vi "Test Process Helper Loop Stopped when Process Stopped.vi"(8 "error in (no error)":errorcluster, 11 "Helper Loop Test In":refnum<class "Process Test.lvclass">) -> (0 "error out":errorcluster, 3 "Helper Loop Test Out":refnum<class "Process Test.lvclass">)   [LabVIEW 2020, in "Process Test.lvclass"]
uses:
  Process Test/Process Test.lvclass
  C:/Program Files (x86)/National Instruments/LabVIEW 2020/vi.lib/Asteme/LUnit/Test Case.lvclass
  Framework/Helper Loop/Helper Loop.lvclass
  <vilib>/Asteme/LUnit/Test Case.lvclass/Test Case.ctl
  <vilib>/Asteme/LUnit/LUnit Assertion Result.lvclass/LUnit Assertion Result.ctl
  Framework/Process/Process.lvclass/Process.ctl
  Support/Event Helpers/Dequeue Event Message by Message.vi
  <vilib>/Asteme/LUnit/Palette/Pass.vi
  <vilib>/Asteme/LUnit/Palette/Fail.vi
  <vilib>/Asteme/LUnit/Variant to string.vi
  <vilib>/Asteme/LUnit/Set Assertion Type.vi
  Framework/Process/Public/Get Lifecycle State.vi
  Framework/Process/Private/SubVIs/Wait for finish.vi
  Framework/Process/Protected/Messaging/Enqueue Message.vi
  Framework/Process/Private/SubVIs/Set Lifecycle State.vi
  <vilib>/Asteme/LUnit/Add test result.vi
  <vilib>/Asteme/LUnit/LUnit Get Test Case.vi
  <vilib>/Asteme/LUnit/LUnit Write Message.vi
  <vilib>/Asteme/LUnit/LUnit Write Description.vi
  <vilib>/Asteme/LUnit/LUnit Write Skipped.vi
  Support/Execution timer.vi
  <vilib>/Asteme/LUnit/LUnit Write Passed.vi
  <vilib>/Asteme/LUnit/LUnit Write Assertion Type.vi
  <vilib>/Utility/error.llb/Clear Errors.vi
  <vilib>/AdvancedString/1D String Array to Delimited String.vi
  <vilib>/Asteme/LUnit/Read Test Case Name.vi
  Support/Event Helpers/Dequeue Event Message.vi
  <vilib>/Asteme/LUnit/Assertion Result/LUnit Get Test Name.vi
  <vilib>/Utility/Data Type/Get Type Information.vi
  <vilib>/Utility/LVClass/Get LV Class Name.vi
  <vilib>/Utility/error.llb/Error Cluster From Error Code.vi
  <vilib>/Asteme/LUnit/LUnit Assertion Result.lvclass
  Framework/Process/Process.lvclass
  <vilib>/Asteme/LUnit/Test Case.lvclass
  Support/Event Helpers/Event Helpers.lvlib
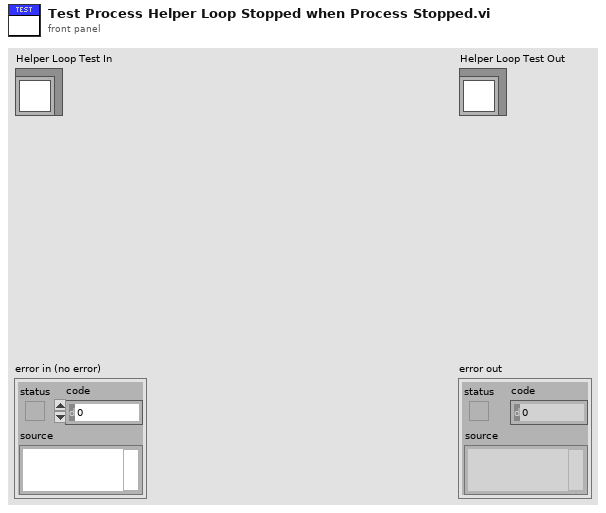
[diagram p1: front panel]
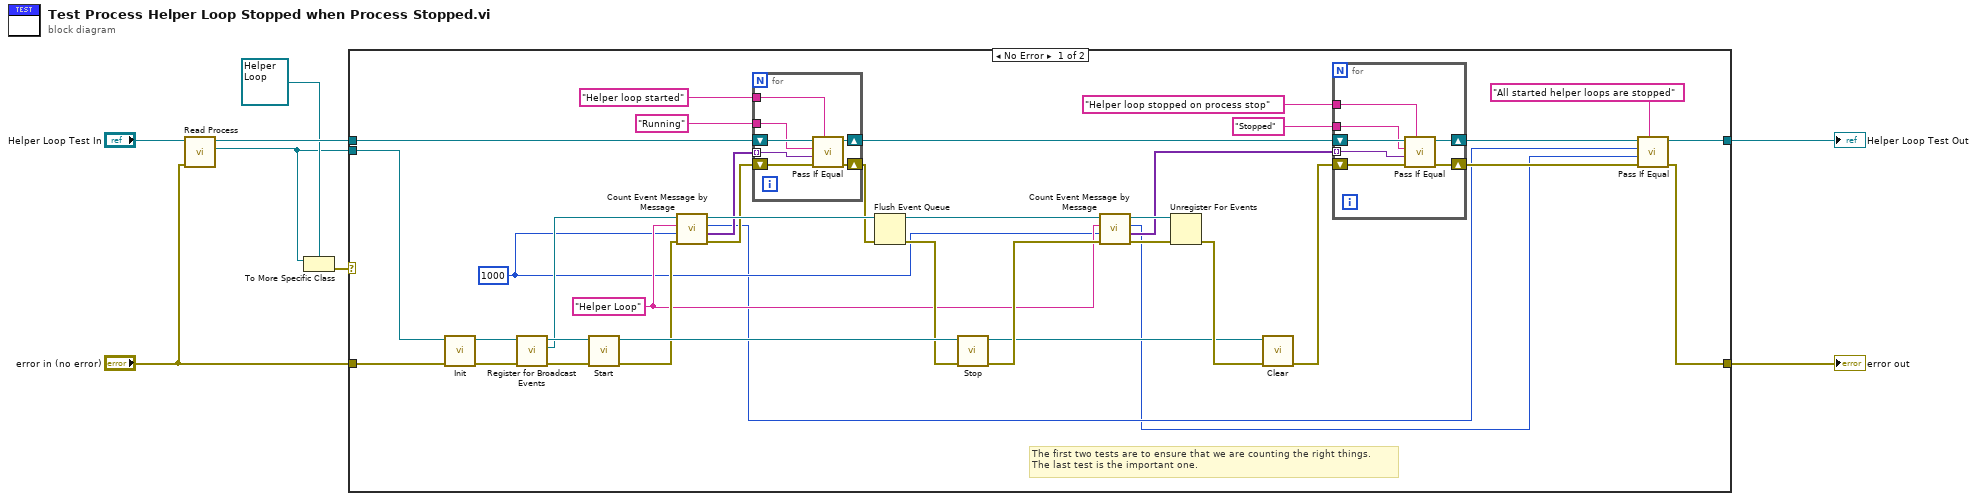
[diagram p0: block diagram]
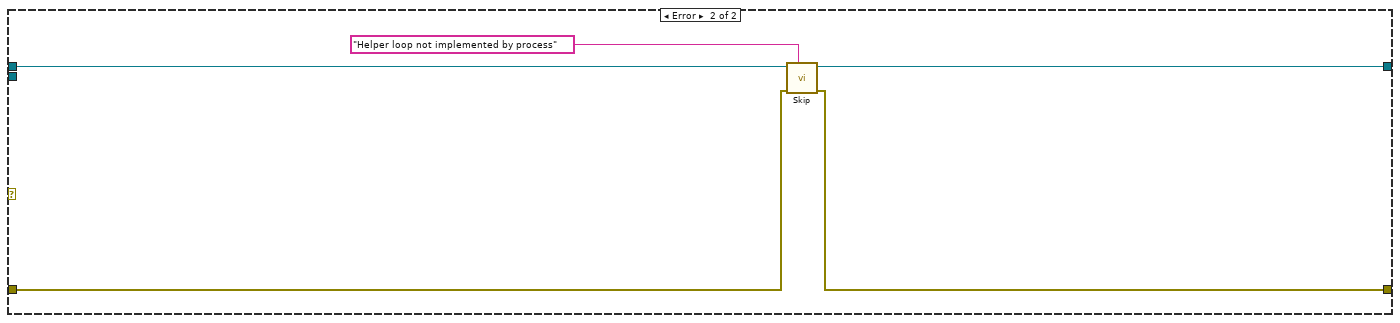
[diagram p2: hidden frame]
diagram:
  n1 = call "Read Process.vi"("error in (no error)"="error in (no error)", "Process Test in"="Helper Loop Test In") -> ("Process.lvclass"=w1:refnum<class "Process.lvclass">, "Process Test out"=w5:refnum<class "Process Test.lvclass">)  [unwired: 7 in, 1 out]
  n2 = To More Specific Class(target class=refnum<class "Helper Loop.lvclass"> refnum ("Helper Loop.lvclass"), reference=w1) -> (error out=w3:errorcluster)  [unwired: 1 in, 1 out]
  n3 = case shown="No Error" w3 {
    tunnel: [w15 w63] -> w8
    tunnel: "error in (no error)" -> [w39 w62]
    tunnel: [w13 w61] -> w7
    tunnel: w5 -> [w25 w64]
    tunnel: w1 -> [w31 _]
    frame No Error {
      w24 = 1000 ("Timeout (-1)")
      w27 = "Helper Loop" ("y")
      # "The first two tests are to ensure that we are counting the right things. \nThe last test is the important one."
      n4 = call-dynamic "Init.vi"("error in (no error)"=w39, "Process In"=w31) -> ("error out"=w44:errorcluster, "Process Out"=w45:refnum<class "Process.lvclass">)  [unwired: 8 in]
      n5 = call-dynamic "Register for Broadcast Events.vi"("error in (no error)"=w44, "Process In"=w45) -> ("error out"=w42:errorcluster, "Event Registration Refnum"=w30:refnum<event-registration>, "Process Out"=w43:refnum<class "Process.lvclass">)  [unwired: 7 in]
      n6 = call "Start.vi"("error in (no error)"=w42, "Process In"=w43) -> ("error out"=w28:errorcluster, "Process Out"=w41:refnum<class "Process.lvclass">)  [unwired: 8 in]
      n7 = call "Count Event Message by Message.vi"("error in (no error)"=w28, "Timeout"=w24, "Message"=w27, "Event Registration Refnum in"=w30) -> ("error out"=w23:errorcluster, "Message Data"=w19:variant[], "Count"=w12:i32, "Event Registration Refnum out"=w29:refnum<event-registration>)  [unwired: 4 in]
      n8 = for {
        tunnel: "Helper loop started" ("Description") -> [w48]
        tunnel: "Running" ("Description") -> [w47]
        shift-right: [w52] -> w26
        shift-left: w25 -> [w51]
        shift-right: [w49] -> w22
        shift-left: w23 -> [w50]
        tunnel: w19 -> [w46] mode=indexing
        n9 = call <vilib>:"Pass If Equal.vi"("Description"=w48, "error in (no error)"=w50, "Actual"=w46, "Expected"=w47, "Test Case In"=w51) -> ("error out"=w49:errorcluster, "Test Case Out"=w52:refnum<class "Process Test.lvclass">)  [unwired: 5 in]
      }
      n10 = Flush Event Queue(0:w29, 3:w22) -> (8:w36:refnum<event-registration>, 11:w35:errorcluster)  [unwired: 4 in, 1 out]
      n11 = call "Stop.vi"("error in (no error)"=w35, "Process In"=w41) -> ("error out"=w34:errorcluster, "Process Out"=w33:refnum<class "Process.lvclass">)  [unwired: 7 in, 1 out]
      n12 = call "Count Event Message by Message.vi"("error in (no error)"=w34, "Timeout"=w24, "Message"=w27, "Event Registration Refnum in"=w36) -> ("error out"=w32:errorcluster, "Message Data"=w18:variant[], "Count"=w11:i32, "Event Registration Refnum out"=w38:refnum<event-registration>)  [unwired: 4 in]
      n13 = Unregister For Events(event registration refnum=w38, error in=w32) -> (error out=w37:errorcluster)
      n14 = call-dynamic "Clear.vi"("error in (no error)"=w37, "Process In"=w33) -> ("error out"=w40:errorcluster)  [unwired: 8 in, 1 out]
      n15 = for {
        tunnel: w18 -> [w56] mode=indexing
        shift-right: [w57] -> w14
        shift-left: w40 -> [w59]
        shift-right: [w58] -> w16
        shift-left: w26 -> [w55]
        tunnel: "Helper loop stopped on process stop" ("Description") -> [w54]
        tunnel: "Stopped" ("Description") -> [w53]
        n16 = call <vilib>:"Pass If Equal.vi"("Description"=w54, "error in (no error)"=w59, "Actual"=w56, "Expected"=w53, "Test Case In"=w55) -> ("error out"=w57:errorcluster, "Test Case Out"=w58:refnum<class "Process Test.lvclass">)  [unwired: 5 in]
      }
      n17 = call <vilib>:"Pass If Equal.vi"("Description"="All started helper loops are stopped", "error in (no error)"=w14, "Actual"=w11, "Expected"=w12, "Test Case In"=w16) -> ("error out"=w13:errorcluster, "Test Case Out"=w15:refnum<class "Process Test.lvclass">)  [unwired: 5 in]
    }
    frame Error {
      n18 = call <vilib>:"Skip.vi"("Description"="Helper loop not implemented by process", "error in (no error)"=w62, "Test Case In"=w64) -> ("error out"=w61:errorcluster, "Test Case Out"=w63:refnum<class "Process Test.lvclass">)  [unwired: 7 in]
    }
  }
  "error out" <- w7
  "Helper Loop Test Out" <- w8
